vi "ApplyConfigurationName.vi"() -> (1 "message name":string)   [LabVIEW 2017, in "ServerComm.lvlib"]
doc: "Returns the following message name: ServerComm.ApplyConfiguration. The NI-developed Controller process handles this message by restarting the device software and writing information to the reboot log about this expected shutdown."
uses:
  <vilib>/addons/InsightCM/Devices/Shared/Common/ServerComm/ServerComm.lvlib
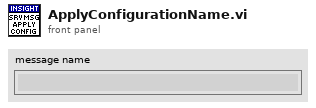
[diagram p1: front panel]
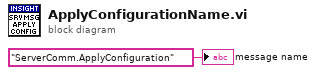
[diagram p0: block diagram]
diagram:
  "message name" <- "ServerComm.ApplyConfiguration" ("ProcessName")
